vi "Move Beam.vi"(11 "Track Point":T1) -> (2 "Next Position Out":T2, 3 "Track Point Out":T1)   [LabVIEW 2023]
uses:
  Cluster_Point.ctl
  Cluster_Tracking point.ctl
  ENUM_Direction_a2.ctl
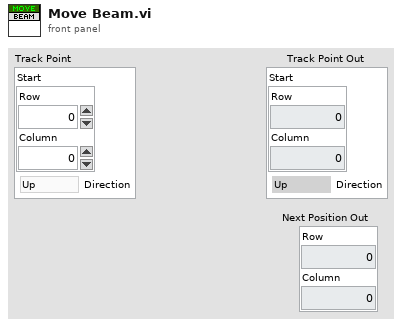
[diagram p1: front panel]
types:
  T1 = typedef "Cluster_Tracking point.ctl" = cluster{"Start":T2, "Direction":T3}
  T2 = typedef "Cluster_Point.ctl" = cluster{"Row":i32, "Column":i32}
  T3 = typedef "ENUM_Direction_a2.ctl" = enum16{"Up", "Left", "Down", "Right", "Up-Down", "Left-Right"}
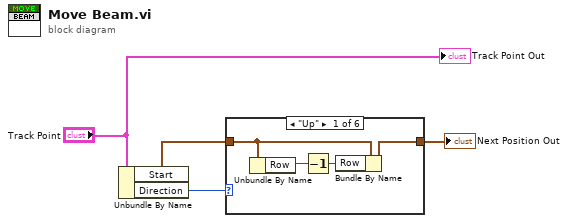
[diagram p0: block diagram]
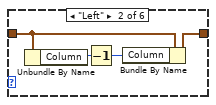
[diagram p2: hidden frame]
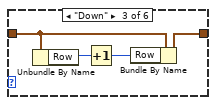
[diagram p3: hidden frame]
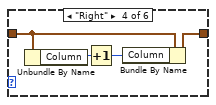
[diagram p4: hidden frame]
diagram:
  n1 = Unbundle By Name("Track Point") -> ("Start"=w2:T2, "Direction"=w3:T3)
  n2 = case shown="\"Up\"" w3 {
    tunnel: w2 -> [w6 w10 w14 w18 w21 w22]
    tunnel: [w5 w9 w13 w17 w21 w22] -> w4
    frame "Up" {
      n3 = Unbundle By Name(w6) -> ("Row"=w8:i32)
      n4 = Decrement(x=w8) -> (x-1=w7:i32)
      n5 = Bundle By Name(cluster=w6, "Row"=w7) -> (w5:T2)
    }
    frame "Left" {
      n6 = Unbundle By Name(w10) -> ("Column"=w12:i32)
      n7 = Decrement(x=w12) -> (x-1=w11:i32)
      n8 = Bundle By Name(cluster=w10, "Column"=w11) -> (w9:T2)
    }
    frame "Down" {
      n9 = Unbundle By Name(w14) -> ("Row"=w16:i32)
      n10 = Increment(x=w16) -> (x+1=w15:i32)
      n11 = Bundle By Name(cluster=w14, "Row"=w15) -> (w13:T2)
    }
    frame "Right" {
      n12 = Unbundle By Name(w18) -> ("Column"=w20:i32)
      n13 = Increment(x=w20) -> (x+1=w19:i32)
      n14 = Bundle By Name(cluster=w18, "Column"=w19) -> (w17:T2)
    }
    frame "Up-Down" {
    }
    frame "Left-Right" {
    }
  }
  "Next Position Out" <- w4
  "Track Point Out" <- "Track Point"
